vi "Programa.vi"() -> ()   [LabVIEW 2016]
panel:
  out "Tiempo":dbl format="%#_5g"
  in  "Stop Button":bool
  in  "Test start":bool
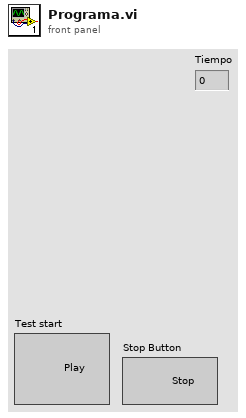
[diagram p1: front panel]
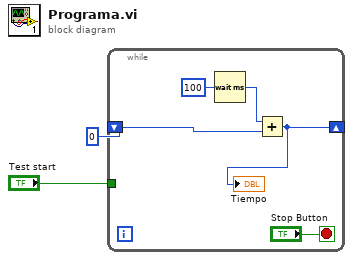
[diagram p0: block diagram]
diagram:
  n1 = while {
    shift-right: [w3] -> _
    shift-left: u32 0 -> [w5]
    tunnel: "Test start" -> [_]
    stop <- "Stop Button" stop-if-true
    n2 = Wait (ms)(milliseconds to wait=u32 100) -> (millisecond timer value=w6:u32)
    n3 = Add(x=w6, y=w5) -> (x+y=w3:u32)
    "Tiempo" <- w3
  }
